vi "Synchronize Module Events.vi"(8 "error in":errorcluster, 9 "Wait for Event Sync?":bool) -> (0 "error out":errorcluster)   [LabVIEW 2018, in "PLC_Launcher.lvlib"]
doc: "Call this VI to ensure the module and its caller have appropriately created and registered for events. This VI should be called after a module's caller registers for events, but before the module's caller's event structure starts. Note that registering for events is optional, but calling this VI must always be done after calling the <b>Start Module.vi</b> for a module.\n\nThis VI must run after the Register for Events function to ensure that no events are missed that are fired by the module after sync occurs. To see an example of the proper wiring pattern, see the \"Start Module: Value Change\" event frame in the API Tester VI for this module.\n_____\nBased on DQMH Project Template 6.0.0.91."
uses:
  PLC_Launcher.lvlib
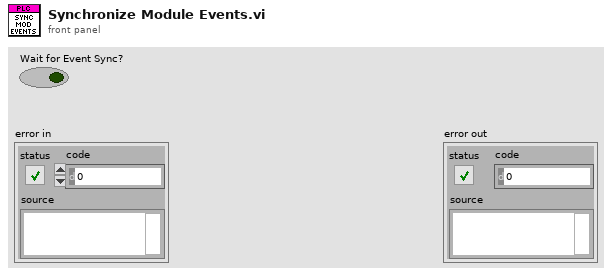
[diagram p1: front panel]
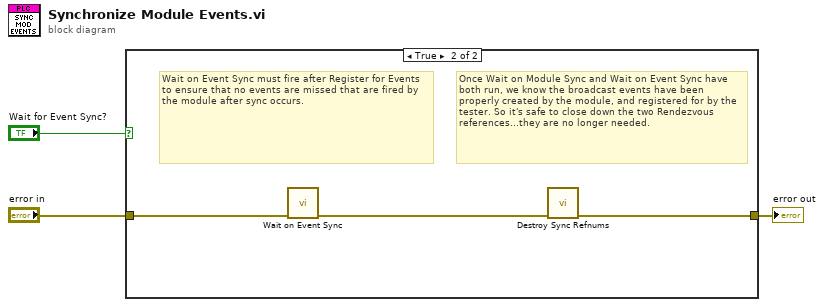
[diagram p0: block diagram]
diagram:
  n1 = case shown="True" "Wait for Event Sync?" {
    tunnel: "error in" -> [w4 w7]
    tunnel: [w4 w5] -> w2
    frame False {
      # "Module was already running, so the sync has already occurred elsewhere."
    }
    frame True {
      # "Once Wait on Module Sync and Wait on Event Sync have both run, we know the broadcast events have been properly created by the module, and registered for by the tester. So it's safe to close down the two Rendezvous references...they are no longer needed."
      # "Wait on Event Sync must fire after Register for Events to ensure that no events are missed that are fired by the module after sync occurs."
      n2 = call "Wait on Event Sync.vi"("error in (no error)"=w7) -> ("error out"=w6:errorcluster)  [unwired: 10 in]
      n3 = call "Destroy Sync Refnums.vi"("error in (no error)"=w6) -> ("error out"=w5:errorcluster)  [unwired: 10 in]
    }
  }
  "error out" <- w2
